vi "AR Drone - Gamepad NavData Video.vi"() -> (2 "Hover?":bool, 3 "Video Stream":picture)   [LabVIEW 2015]
doc: "Example demonstrating how to control the AR Drone with a joystick or gamepad and simultaneously receive navigation and video data."
uses:
  <vilib>/LVH/AR Drone Toolkit/Decode NavData/Typedefs/NavData Demo.ctl
  <vilib>/LVH/AR Drone Toolkit/Type Defs/Flight Animations.ctl
  <vilib>/Utility/inputDevices.llb/closeJoystick.vi
  <vilib>/LVH/AR Drone Toolkit/AR Drone.lvlib
panel:
  out "Pitching speed":dbl
  out "Yawing speed":sgl
  out "Vertical speed":sgl
  in  "Autopilot":bool
  in  "Stop FSM":bool
  in  "Reset":bool
  in  "Start":bool
  in  "Desired yaw":i16
  in  "Restart":bool
  in  "State":i8=1 min=1 max=33 step=1
  out "Downward loop":i8
  out "Snake loop":i8
  out "Upward loop":i8
  out "Current yaw":sgl
  out "Height":i16
  in  "Yaw speed":sgl(slide) min=-1 max=1 scale=-1.0..1.0
  in  "V speed":sgl(slide) min=-1 max=1 scale=-1.0..1.0
  in  "Pitch":sgl(slide) min=-1 max=1 scale=-1.0..1.0
  in  "Roll":sgl(slide) min=-1 max=1 scale=-1.0..1.0
  in  "display/gamepad":bool
  out "Gamepad Output":T1
  in  "Flight Animations":T2 items=["PHI_M30_DEG", "PHI_30_DEG", "THETA_M30_DEG", "THETA_30_DEG", "THETA_20DEG_YAW_200DEG", "THETA_20DEG_YAW_M2000DEG", "TURNAROUND", "TURNAROUND_GODOWN", "YAW_SHAKE", "YAW_DANCE", "PHI_DANCE", "THETA_DANCE", "VZ_DANCE", "WAVE", "PHI_THETA_MIXED", "DOUBLE_PHI_THETA_MIXED", "FLIP_AHEAD", "FLIP_BEHIND", "FLIP_LEFT", "FLIP_RIGHT", "NB_ANIM_MAYDAY"]
  out "NavData Out":T3
  out "Battery Remaining":dbl(slide) scale=0.0..100.0
  out "Axes Output":T4 {"Vertical Speed" scale=-1.0..1.0; "Yaw Speed" scale=-1.0..1.0; "Pitch" scale=-1.0..1.0; "Roll" scale=-1.0..1.0}
  in  "stop":bool
  # "Xbox Controller:\nLeft stick L/R - Roll\nLeft stick D/U - Pitch\nL/R Triggers - Vertical Speed\nRight stick L/R - Yaw Speed"
  # "Xbox Controller:\nA - take off\nB - emergency\nX - hover\nStart - Stop"
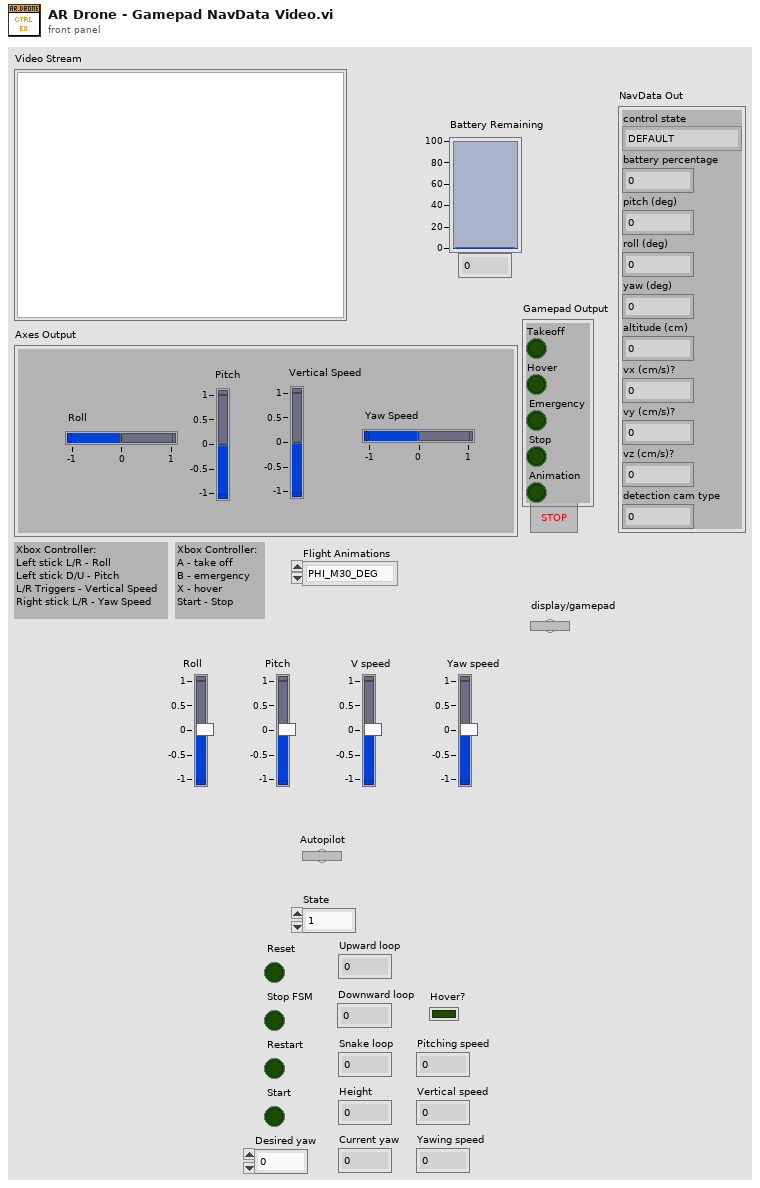
[diagram p1: front panel]
types:
  T1 = cluster{"Takeoff":bool, "Hover":bool, "Emergency":bool, "Stop":bool, "Animation":bool}
  T2 = typedef "AR Drone.lvlib/Flight Animations.ctl" = u16
  T3 = typedef "AR Drone.lvlib/NavData Demo.ctl" = cluster{"control state":enum32{"DEFAULT", "INIT", "LANDING", "FLYING", "HOVERING", "TEST", "TRANS_TAKEOFF", "TRANS_GOTOFIX", "TRANS_LANDING"}, "battery percentage":u32, "pitch (deg)":sgl, "roll (deg)":sgl, "yaw (deg)":sgl, "altitude (cm)":u32, "vx (cm/s)?":sgl, "vy (cm/s)?":sgl, "vz (cm/s)?":sgl, "detection cam type":u32}
  T4 = cluster{"Roll":dbl, "Pitch":dbl, "Vertical Speed":dbl, "Yaw Speed":dbl}
  T5 = typedef "AR Drone.lvlib/AR Drone Resource.ctl" = cluster{"UDP Control Connection":refnum<k16>, "UDP NavData Connection":refnum<k16>, "UDP Video Connection (Drone 1.0)":refnum<k16>, "TCP Video Connection (Drone 2.0)":refnum<k5>, "TCP Control Port Connection":refnum<k5>, "Drone IP address":string, "Drone Command Port":u16, "Drone NavData Port":u16, "Drone Vid Stream Port":u16, "Drone TCP Control Port":u16, "Home IP address":string, "Home Command Port":u16, "Home NavData Port":u16, "Home Vid Stream Port":u16, "Drone Version":i32}
  T6 = cluster{"Roll":sgl, "Pitch":sgl, "Vertical Speed":sgl, "Yaw Speed":sgl}
  T7 = cluster{"Roll":sgl, "Pitch":sgl, "V speed":sgl, "Yaw speed":sgl}
  T8 = cluster{"Yawing speed":sgl, "Pitching speed":dbl, "Vertical speed":sgl, "Yawing speed":sgl}
  T9 = cluster{"Roll":sgl, "Pitching speed":dbl, "V speed":sgl, "Yaw speed":sgl}
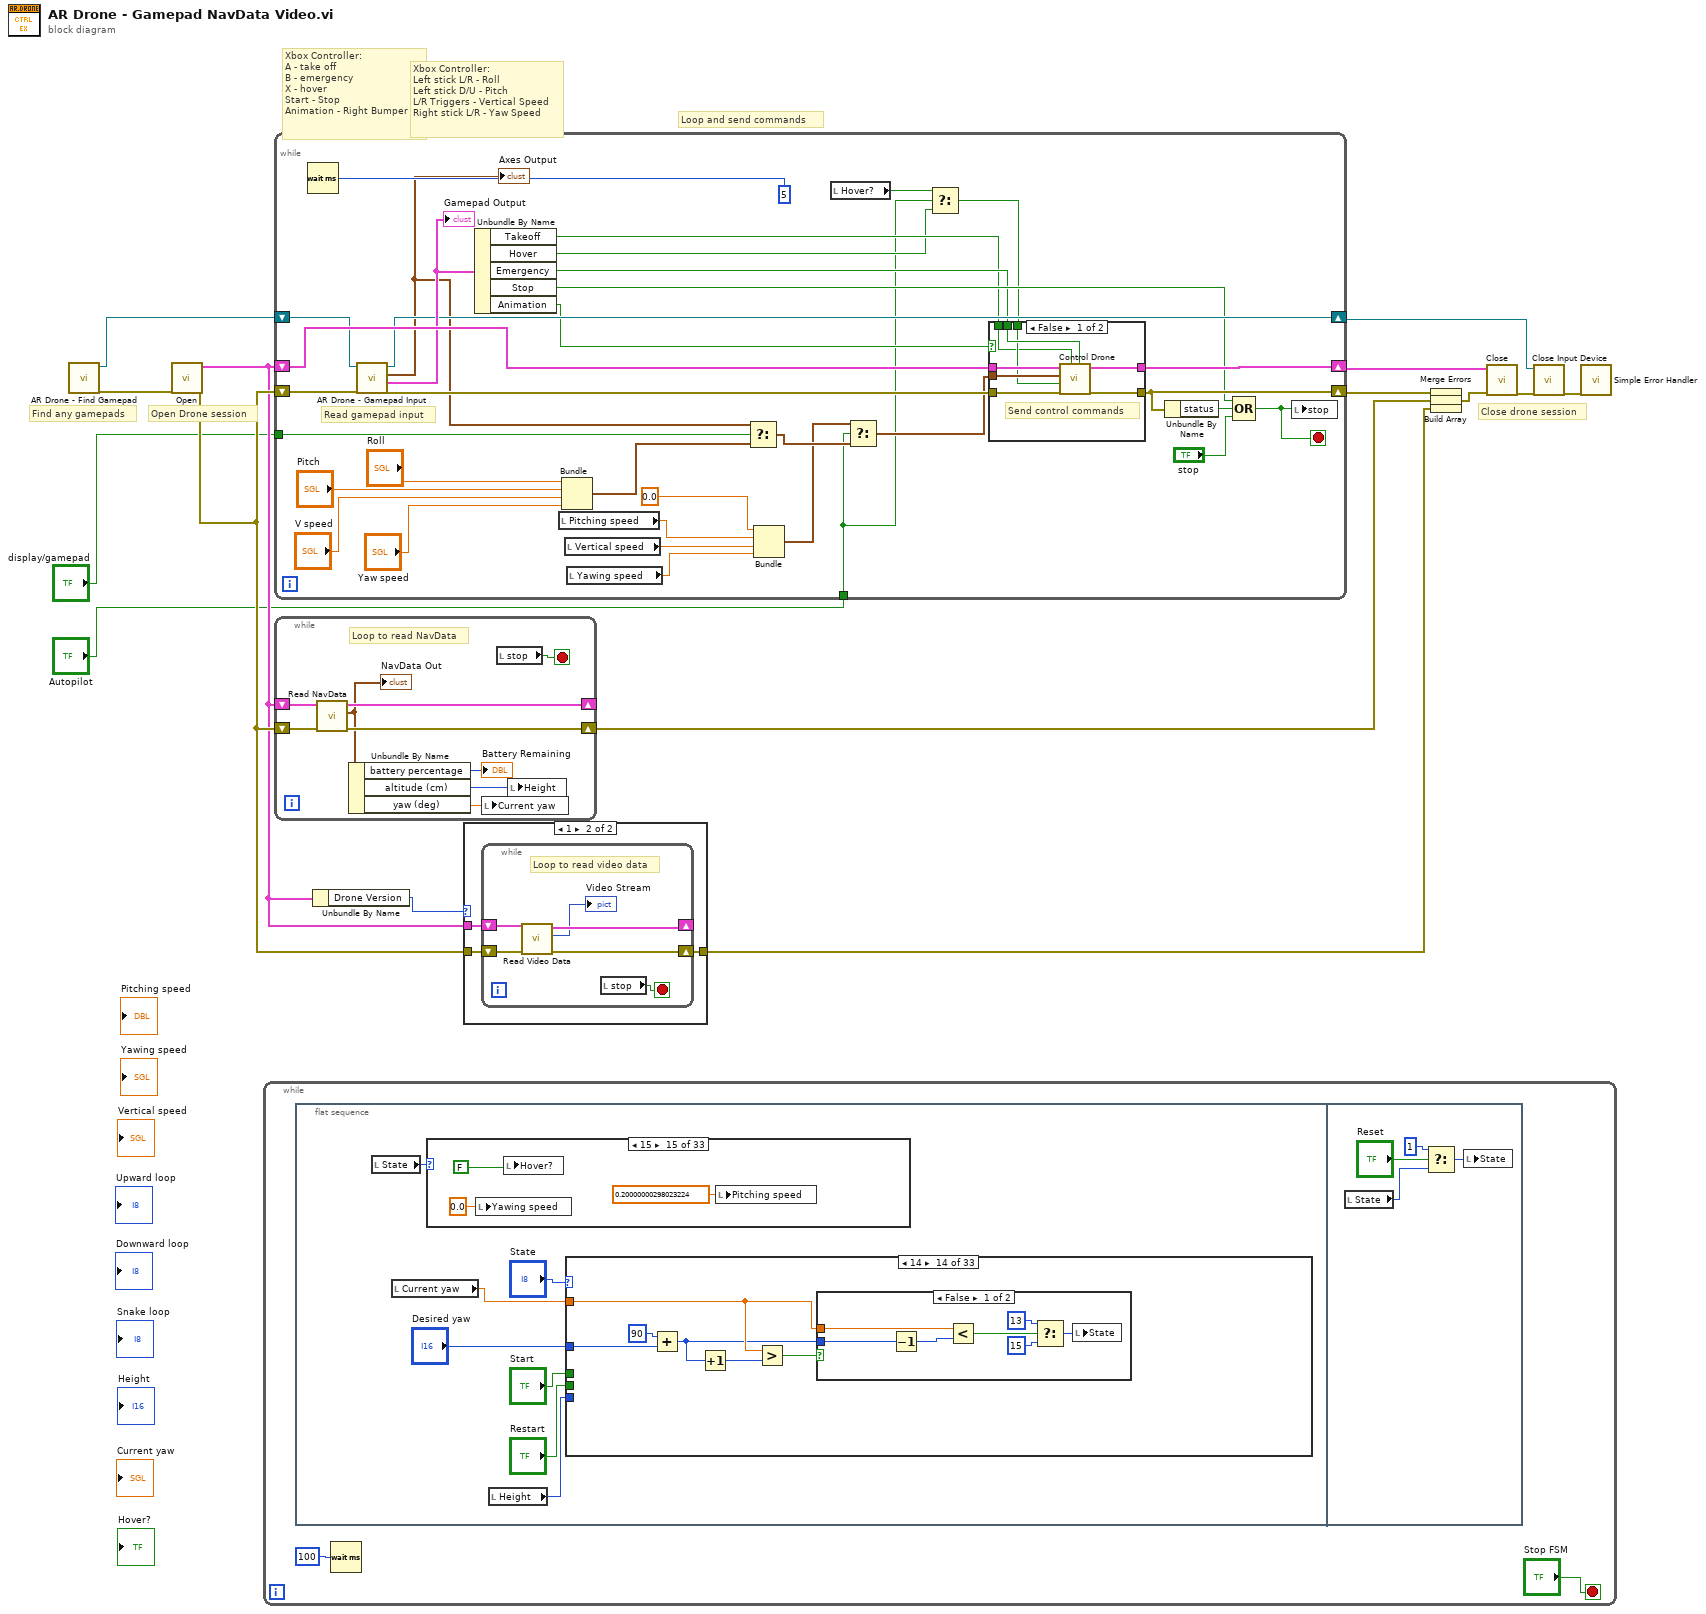
[diagram p0: block diagram]
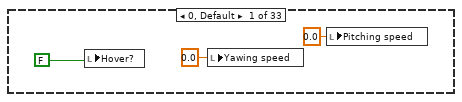
[diagram p2: hidden frame]
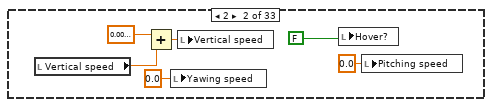
[diagram p3: hidden frame]
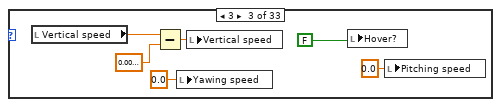
[diagram p4: hidden frame]
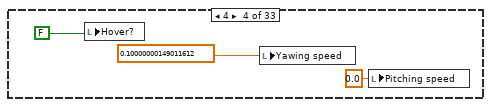
[diagram p5: hidden frame]
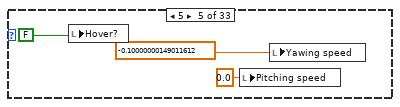
[diagram p6: hidden frame]
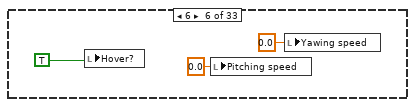
[diagram p7: hidden frame]
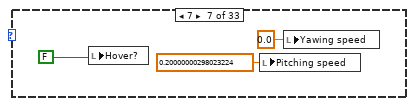
[diagram p8: hidden frame]
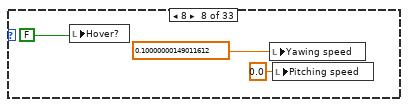
[diagram p9: hidden frame]
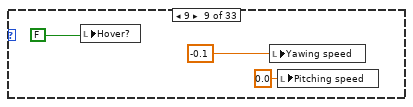
[diagram p10: hidden frame]
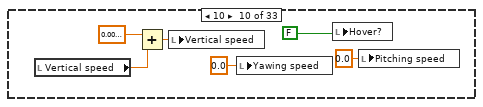
[diagram p11: hidden frame]
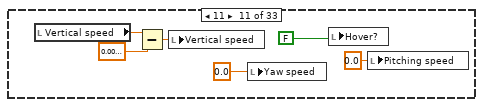
[diagram p12: hidden frame]
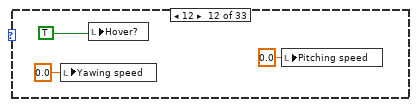
[diagram p13: hidden frame]
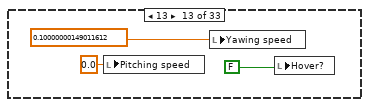
[diagram p14: hidden frame]
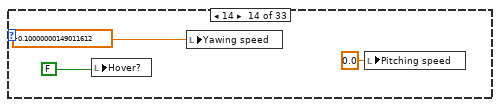
[diagram p15: hidden frame]
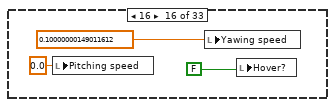
[diagram p16: hidden frame]
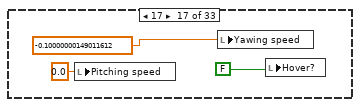
[diagram p17: hidden frame]
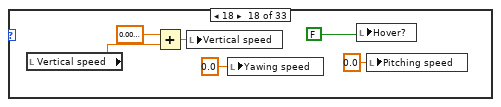
[diagram p18: hidden frame]
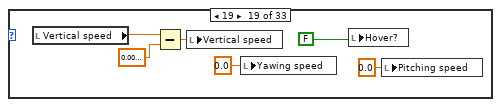
[diagram p19: hidden frame]
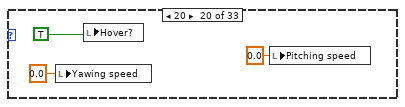
[diagram p20: hidden frame]
diagram:
  # "Loop and send commands"
  # "Close drone session"
  # "Open Drone session"
  # "Find any gamepads"
  # "Xbox Controller:\nLeft stick L/R - Roll\nLeft stick D/U - Pitch\nL/R Triggers - Vertical Speed\nRight stick L/R - Yaw Speed"
  # "Xbox Controller:\nA - take off\nB - emergency\nX - hover\nStart - Stop\nAnimation - Right Bumper"
  n1 = call "AR Drone - Find Gamepad.vi"() -> ("error out"=w11:errorcluster, "Refnum out"=w12:refnum<k1>)  [unwired: 10 in]
  n2 = call <vilib>:"Open.vi"("error in (no error)"=w11) -> ("error out"=w6:errorcluster, "AR Drone Resource"=w4:T5)  [unwired: 9 in]
  n3 = while {
    stop <- "Stop FSM" stop-if-true
    n4 = flat-sequence {
      frame #0 {
        n5 = local read "State"() -> (w20:i8)
        n6 = local read "Current yaw"() -> (w23:sgl)
        n7 = case shown="15" w20 {
          frame 0, Default {
            n8 = local write "Hover?"(FALSE) -> ()
            n9 = local write "Yawing speed"(sgl 0.0 ("Yawing speed")) -> ()
            n10 = local write "Pitching speed"(sgl 0.0 ("Yawing speed")) -> ()
          }
          frame 2 {
            n11 = local read "Vertical speed"() -> (w33:sgl)
            n12 = Add(x=sgl 0.01, y=w33) -> (x+y=w34:sgl)
            n13 = local write "Yawing speed"(sgl 0.0 ("Yawing speed")) -> ()
            n14 = local write "Vertical speed"(w34) -> ()
            n15 = local write "Hover?"(FALSE) -> ()
            n16 = local write "Pitching speed"(sgl 0.0 ("Yawing speed")) -> ()
          }
          frame 3 {
            n17 = local read "Vertical speed"() -> (w39:sgl)
            n18 = Subtract(x=w39, y=sgl 0.01 ("x")) -> (x-y=w40:sgl)
            n19 = local write "Yawing speed"(sgl 0.0 ("Yawing speed")) -> ()
            n20 = local write "Vertical speed"(w40) -> ()
            n21 = local write "Hover?"(FALSE) -> ()
            n22 = local write "Pitching speed"(sgl 0.0 ("Yawing speed")) -> ()
          }
          frame 4 {
            n23 = local write "Hover?"(FALSE) -> ()
            n24 = local write "Yawing speed"(sgl 0.1 ("Yawing speed")) -> ()
            n25 = local write "Pitching speed"(sgl 0.0 ("Yawing speed")) -> ()
          }
          frame 5 {
            n26 = local write "Hover?"(FALSE) -> ()
            n27 = local write "Pitching speed"(sgl 0.0 ("Yawing speed")) -> ()
            n28 = local write "Yawing speed"(sgl -0.1 ("Yawing speed")) -> ()
          }
          frame 6 {
            n29 = local write "Hover?"(TRUE) -> ()
            n30 = local write "Pitching speed"(sgl 0.0 ("Yawing speed")) -> ()
            n31 = local write "Yawing speed"(sgl 0.0 ("Yawing speed")) -> ()
          }
          frame 7 {
            n32 = local write "Hover?"(FALSE) -> ()
            n33 = local write "Pitching speed"(sgl 0.2 ("Yawing speed")) -> ()
            n34 = local write "Yawing speed"(sgl 0.0 ("Yawing speed")) -> ()
          }
          frame 8 {
            n35 = local write "Hover?"(FALSE) -> ()
            n36 = local write "Yawing speed"(sgl 0.1 ("Yawing speed")) -> ()
            n37 = local write "Pitching speed"(sgl 0.0 ("Yawing speed")) -> ()
          }
          frame 9 {
            n38 = local write "Hover?"(FALSE) -> ()
            n39 = local write "Yawing speed"(-0.1 ("Yawing speed")) -> ()
            n40 = local write "Pitching speed"(sgl 0.0 ("Yawing speed")) -> ()
          }
          frame 10 {
            n41 = local read "Vertical speed"() -> (w64:sgl)
            n42 = Add(x=sgl 0.01, y=w64) -> (x+y=w63:sgl)
            n43 = local write "Vertical speed"(w63) -> ()
            n44 = local write "Yawing speed"(sgl 0.0 ("Yawing speed")) -> ()
            n45 = local write "Hover?"(FALSE) -> ()
            n46 = local write "Pitching speed"(sgl 0.0 ("Yawing speed")) -> ()
          }
          frame 11 {
            n47 = local read "Vertical speed"() -> (w69:sgl)
            n48 = Subtract(x=w69, y=sgl 0.01) -> (x-y=w70:sgl)
            n49 = local write "Vertical speed"(w70) -> ()
            n50 = local write "Yaw speed"(sgl 0.0 ("Yawing speed")) -> ()
            n51 = local write "Hover?"(FALSE) -> ()
            n52 = local write "Pitching speed"(sgl 0.0 ("Yawing speed")) -> ()
          }
          frame 12 {
            n53 = local write "Yawing speed"(sgl 0.0 ("Yawing speed")) -> ()
            n54 = local write "Hover?"(TRUE) -> ()
            n55 = local write "Pitching speed"(sgl 0.0 ("Yawing speed")) -> ()
          }
          frame 13 {
            n56 = local write "Pitching speed"(sgl 0.0 ("Yawing speed")) -> ()
            n57 = local write "Yawing speed"(sgl 0.1 ("Yawing speed")) -> ()
            n58 = local write "Hover?"(FALSE) -> ()
          }
          frame 14 {
            n59 = local write "Hover?"(FALSE) -> ()
            n60 = local write "Yawing speed"(sgl -0.1 ("Yawing speed")) -> ()
            n61 = local write "Pitching speed"(sgl 0.0 ("Yawing speed")) -> ()
          }
          frame 15 {
            n62 = local write "Yawing speed"(sgl 0.0 ("Yawing speed")) -> ()
            n63 = local write "Hover?"(FALSE) -> ()
            n64 = local write "Pitching speed"(sgl 0.2 ("Yawing speed")) -> ()
          }
          frame 16 {
            n65 = local write "Pitching speed"(sgl 0.0 ("Yawing speed")) -> ()
            n66 = local write "Yawing speed"(sgl 0.1 ("Yawing speed")) -> ()
            n67 = local write "Hover?"(FALSE) -> ()
          }
          frame 17 {
            n68 = local write "Pitching speed"(sgl 0.0 ("Yawing speed")) -> ()
            n69 = local write "Yawing speed"(sgl -0.1 ("Yawing speed")) -> ()
            n70 = local write "Hover?"(FALSE) -> ()
          }
          frame 18 {
            n71 = local read "Vertical speed"() -> (w94:sgl)
            n72 = Add(x=sgl 0.01, y=w94) -> (x+y=w93:sgl)
            n73 = local write "Vertical speed"(w93) -> ()
            n74 = local write "Yawing speed"(sgl 0.0 ("Yawing speed")) -> ()
            n75 = local write "Hover?"(FALSE) -> ()
            n76 = local write "Pitching speed"(sgl 0.0 ("Yawing speed")) -> ()
          }
          frame 19 {
            n77 = local read "Vertical speed"() -> (w99:sgl)
            n78 = Subtract(x=w99, y=sgl 0.01) -> (x-y=w100:sgl)
            n79 = local write "Vertical speed"(w100) -> ()
            n80 = local write "Yawing speed"(sgl 0.0 ("Yawing speed")) -> ()
            n81 = local write "Hover?"(FALSE) -> ()
            n82 = local write "Pitching speed"(sgl 0.0 ("Yawing speed")) -> ()
          }
          frame 20 {
            n83 = local write "Yawing speed"(sgl 0.0 ("Yawing speed")) -> ()
            n84 = local write "Hover?"(TRUE) -> ()
            n85 = local write "Pitching speed"(sgl 0.0 ("Yawing speed")) -> ()
          }
          frame 21 {
            n86 = local write "Yawing speed"(sgl 0.0 ("Yawing speed")) -> ()
            n87 = local write "Hover?"(FALSE) -> ()
            n88 = local write "Pitching speed"(sgl 0.0 ("Yawing speed")) -> ()
          }
          frame 22 {
            n89 = local write "Pitching speed"(sgl 0.0 ("Yawing speed")) -> ()
            n90 = local write "Yawing speed"(sgl 0.1 ("Yawing speed")) -> ()
            n91 = local write "Hover?"(FALSE) -> ()
          }
          frame 23 {
            n92 = local write "Pitching speed"(sgl 0.0 ("Yawing speed")) -> ()
            n93 = local write "Yawing speed"(sgl -0.1 ("Yawing speed")) -> ()
            n94 = local write "Hover?"(FALSE) -> ()
          }
          frame 24 {
            n95 = local read "Vertical speed"() -> (w118:sgl)
            n96 = Add(x=sgl 0.01, y=w118) -> (x+y=w117:sgl)
            n97 = local write "Vertical speed"(w117) -> ()
            n98 = local write "Yawing speed"(sgl 0.0 ("Yawing speed")) -> ()
            n99 = local write "Hover?"(FALSE) -> ()
            n100 = local write "Pitching speed"(sgl 0.0 ("Yawing speed")) -> ()
          }
          frame 25 {
            n101 = local read "Vertical speed"() -> (w123:sgl)
            n102 = Subtract(x=w123, y=sgl 0.01) -> (x-y=w124:sgl)
            n103 = local write "Vertical speed"(w124) -> ()
            n104 = local write "Yawing speed"(sgl 0.0 ("Yawing speed")) -> ()
            n105 = local write "Hover?"(FALSE) -> ()
            n106 = local write "Pitching speed"(sgl 0.0 ("Yawing speed")) -> ()
          }
          frame 26 {
            n107 = local write "Yawing speed"(sgl 0.0 ("Yawing speed")) -> ()
            n108 = local write "Hover?"(TRUE) -> ()
            n109 = local write "Pitching speed"(sgl 0.0 ("Yawing speed")) -> ()
          }
          frame 27 {
            n110 = local write "Pitching speed"(sgl 0.0 ("Yawing speed")) -> ()
            n111 = local write "Yawing speed"(sgl 0.1 ("Yawing speed")) -> ()
            n112 = local write "Hover?"(FALSE) -> ()
          }
          frame 28 {
            n113 = local write "Pitching speed"(sgl 0.0 ("Yawing speed")) -> ()
            n114 = local write "Yawing speed"(sgl -0.1 ("Yawing speed")) -> ()
            n115 = local write "Hover?"(FALSE) -> ()
          }
          frame 29 {
            n116 = local write "Yawing speed"(sgl 0.0 ("Yawing speed")) -> ()
            n117 = local write "Hover?"(FALSE) -> ()
            n118 = local write "Pitching speed"(sgl 0.2 ("Yawing speed")) -> ()
          }
          frame 30 {
            n119 = local write "Pitching speed"(sgl 0.0 ("Yawing speed")) -> ()
            n120 = local write "Yawing speed"(sgl 0.1 ("Yawing speed")) -> ()
            n121 = local write "Hover?"(FALSE) -> ()
          }
          frame 31 {
            n122 = local write "Pitching speed"(sgl 0.0 ("Yawing speed")) -> ()
            n123 = local write "Yawing speed"(sgl -0.1 ("Yawing speed")) -> ()
            n124 = local write "Hover?"(FALSE) -> ()
          }
          frame 32 {
            n125 = local write "Yawing speed"(sgl 0.0 ("Yawing speed")) -> ()
            n126 = local write "Hover?"(TRUE) -> ()
            n127 = local write "Pitching speed"(sgl 0.0 ("Yawing speed")) -> ()
          }
          frame 33 {
            n128 = local write "Yawing speed"(sgl 0.0 ("Yawing speed")) -> ()
            n129 = local write "Hover?"(FALSE) -> ()
            n130 = local write "Pitching speed"(sgl 0.0 ("Yawing speed")) -> ()
          }
        }
        n131 = local read "Height"() -> (w24:i16)
        n132 = case shown="14" "State" {
          tunnel: "Start" -> [w152 _ _ _ _ _ _ _ _ _ _ _ _ _ _ _ _ _ _ _ _ _ _ _ _ _ _ _ _ _ _ _ _]
          tunnel: w24 -> [_ w156 w166 _ _ _ _ _ _ w226 w236 _ _ _ _ _ _ w309 w319 _ _ _ _ w359 w369 _ _ _ _ _ _ _ _]
          tunnel: w23 -> [_ _ _ w178 w189 _ _ w203 w215 _ _ _ w255 w269 _ w281 w295 _ _ _ _ w331 w345 _ _ _ w385 w399 _ w415 w429 _ _]
          tunnel: "Desired yaw" -> [_ _ _ w176 w188 _ _ w202 w214 _ _ _ w252 w268 _ w282 w296 _ _ _ _ w332 w346 _ _ _ w386 w400 _ w414 w428 _ _]
          tunnel: "Restart" -> [_ _ _ _ _ _ _ _ _ _ _ _ _ _ _ _ _ _ _ _ _ _ _ _ _ _ _ _ _ _ _ _ w453]
          frame Default {
            n133 = local write "Downward loop"(i8 5 ("pic loop 2")) -> ()
            n134 = Select(t=i8 2, s=w152, f=i8 1) -> (s? t:f=w155:i8)
            n135 = local write "Upward loop"(i8 5 ("pic loop")) -> ()
            n136 = local write "Snake loop"(i8 3 ("snake loop")) -> ()
            n137 = local write "State"(w155) -> ()
          }
          frame 2 {
            n138 = Greater?(x=w156, y=i16 152) -> (0:w157:bool)
            n139 = case shown="False" w157 {
              tunnel: w156 -> [w164 _]
              frame False {
                n140 = Less?(x=w164, y=i16 148) -> (x < y?=w162:bool)
                n141 = Select(t=i8 2, s=w162, f=i8 4) -> (s? t:f=w159:i8)
                n142 = local write "State"(w159) -> ()
              }
              frame True {
                n143 = local write "State"(i8 3 ("state")) -> ()
              }
            }
          }
          frame 3 {
            n144 = Greater?(x=w166, y=i16 152) -> (0:w168:bool)
            n145 = case shown="True" w168 {
              tunnel: w166 -> [w174 _]
              frame False {
                n146 = Less?(x=w174, y=i16 148) -> (x < y?=w172:bool)
                n147 = Select(t=i8 2, s=w172, f=i8 4) -> (s? t:f=w169:i8)
                n148 = local write "State"(w169) -> ()
              }
              frame True {
                n149 = local write "State"(i8 3 ("state")) -> ()
              }
            }
          }
          frame 4 {
            n150 = Increment(x=w176) -> (x+1=w177:i16)
            n151 = Greater?(x=w178, y=w177) -> (0:w179:bool)
            n152 = case shown="True" w179 {
              tunnel: w178 -> [w186 _]
              tunnel: w176 -> [w180 _]
              frame False {
                n153 = Decrement(x=w180) -> (x-1=w181:i16)
                n154 = Less?(x=w186, y=w181) -> (x < y?=w185:bool)
                n155 = Select(t=i8 4, s=w185, f=i8 6) -> (s? t:f=w182:i8)
                n156 = local write "State"(w182) -> ()
              }
              frame True {
                n157 = local write "State"(i8 5 ("state")) -> ()
              }
            }
          }
          frame 5 {
            n158 = Increment(x=w188) -> (x+1=w191:i16)
            n159 = Greater?(x=w189, y=w191) -> (0:w190:bool)
            n160 = case shown="False" w190 {
              tunnel: w189 -> [w198 _]
              tunnel: w188 -> [w192 _]
              frame False {
                n161 = Decrement(x=w192) -> (x-1=w193:i16)
                n162 = Less?(x=w198, y=w193) -> (x < y?=w197:bool)
                n163 = Select(t=i8 4, s=w197, f=i8 6) -> (s? t:f=w194:i8)
                n164 = local write "State"(w194) -> ()
              }
              frame True {
                n165 = local write "State"(i8 5 ("state")) -> ()
              }
            }
          }
          frame 6 {
            n166 = flat-sequence {
              frame #0 {
                n167 = call "Time Delay"() -> ()  [unwired: 11 in, 1 out]
              }
              frame #1 {
                n168 = local write "State"(i8 7 ("state")) -> ()
              }
            }
          }
          frame 7 {
            n169 = flat-sequence {
              frame #0 {
                n170 = call "Time Delay2"() -> ()  [unwired: 11 in, 1 out]
              }
              frame #1 {
                n171 = local write "State"(i8 8 ("state")) -> ()
              }
            }
          }
          frame 8 {
            n172 = Increment(x=w202) -> (x+1=w204:i16)
            n173 = Greater?(x=w203, y=w204) -> (0:w205:bool)
            n174 = case shown="False" w205 {
              tunnel: w203 -> [w212 _]
              tunnel: w202 -> [w206 _]
              frame False {
                n175 = Decrement(x=w206) -> (x-1=w207:i16)
                n176 = Less?(x=w212, y=w207) -> (x < y?=w211:bool)
                n177 = Select(t=i8 8, s=w211, f=i8 10) -> (s? t:f=w208:i8)
                n178 = local write "State"(w208) -> ()
              }
              frame True {
                n179 = local write "State"(i8 9 ("state")) -> ()
              }
            }
          }
          frame 9 {
            n180 = Increment(x=w214) -> (x+1=w217:i16)
            n181 = Greater?(x=w215, y=w217) -> (0:w216:bool)
            n182 = case shown="True" w216 {
              tunnel: w215 -> [w224 _]
              tunnel: w214 -> [w218 _]
              frame False {
                n183 = Decrement(x=w218) -> (x-1=w219:i16)
                n184 = Less?(x=w224, y=w219) -> (x < y?=w223:bool)
                n185 = Select(t=i8 8, s=w223, f=i8 10) -> (s? t:f=w220:i8)
                n186 = local write "State"(w220) -> ()
              }
              frame True {
                n187 = local write "State"(i8 9 ("state")) -> ()
              }
            }
          }
          frame 10 {
            n188 = Greater?(x=w226, y=i16 152) -> (0:w227:bool)
            n189 = case shown="False" w227 {
              tunnel: w226 -> [w234 _]
              frame False {
                n190 = Less?(x=w234, y=i16 148) -> (x < y?=w232:bool)
                n191 = Select(t=i8 10, s=w232, f=i8 12) -> (s? t:f=w229:i8)
                n192 = local write "State"(w229) -> ()
              }
              frame True {
                n193 = local write "State"(i8 11 ("state")) -> ()
              }
            }
          }
          frame 11 {
            n194 = Greater?(x=w236, y=i16 152) -> (0:w238:bool)
            n195 = case shown="False" w238 {
              tunnel: w236 -> [w244 _]
              frame False {
                n196 = Less?(x=w244, y=i16 148) -> (x < y?=w242:bool)
                n197 = Select(t=i8 10, s=w242, f=i8 12) -> (s? t:f=w239:i8)
                n198 = local write "State"(w239) -> ()
              }
              frame True {
                n199 = local write "State"(i8 11 ("state")) -> ()
              }
            }
          }
          frame 12 {
            n200 = flat-sequence {
              frame #0 {
                n201 = call "Time Delay3"() -> ()  [unwired: 11 in, 1 out]
              }
              frame #1 {
                n202 = local read "Upward loop"() -> (w250:i8)
                n203 = Decrement(x=w250) -> (x-1=w251:i8)
                n204 = local write "Upward loop"(w251) -> ()
                n205 = Equal To 0?(x=w251) -> (x = 0?=w246:bool)
                n206 = Select(t=i8 13, s=w246, f=i8 7) -> (s? t:f=w249:i8)
                n207 = local write "State"(w249) -> ()
              }
            }
          }
          frame 13 {
            n208 = Add(x=i16 90, y=w252) -> (x+y=w253:i16)
            n209 = Increment(x=w253) -> (x+1=w257:i16)
            n210 = Greater?(x=w255, y=w257) -> (0:w256:bool)
            n211 = case shown="True" w256 {
              tunnel: w255 -> [w264 _]
              tunnel: w253 -> [w258 _]
              frame False {
                n212 = Decrement(x=w258) -> (x-1=w259:i16)
                n213 = Less?(x=w264, y=w259) -> (x < y?=w263:bool)
                n214 = Select(t=i8 13, s=w263, f=i8 15) -> (s? t:f=w260:i8)
                n215 = local write "State"(w260) -> ()
              }
              frame True {
                n216 = local write "State"(i8 14 ("state")) -> ()
              }
            }
          }
          frame 14 {
            n217 = Add(x=i16 90, y=w268) -> (x+y=w267:i16)
            n218 = Increment(x=w267) -> (x+1=w270:i16)
            n219 = Greater?(x=w269, y=w270) -> (0:w271:bool)
            n220 = case shown="False" w271 {
              tunnel: w269 -> [w278 _]
              tunnel: w267 -> [w272 _]
              frame False {
                n221 = Decrement(x=w272) -> (x-1=w273:i16)
                n222 = Less?(x=w278, y=w273) -> (x < y?=w277:bool)
                n223 = Select(t=i8 13, s=w277, f=i8 15) -> (s? t:f=w274:i8)
                n224 = local write "State"(w274) -> ()
              }
              frame True {
                n225 = local write "State"(i8 14 ("state")) -> ()
              }
            }
          }
          frame 15 {
            n226 = flat-sequence {
              frame #0 {
                n227 = call "Time Delay4"() -> ()  [unwired: 11 in, 1 out]
              }
              frame #1 {
                n228 = local write "State"(i8 16 ("state")) -> ()
              }
            }
          }
          frame 16 {
            n229 = Add(x=i16 180, y=w282) -> (x+y=w286:i16)
            n230 = Increment(x=w286) -> (x+1=w283:i16)
            n231 = Greater?(x=w281, y=w283) -> (0:w284:bool)
            n232 = case shown="True" w284 {
              tunnel: w281 -> [w293 _]
              tunnel: w286 -> [w287 _]
              frame False {
                n233 = Decrement(x=w287) -> (x-1=w288:i16)
                n234 = Less?(x=w293, y=w288) -> (x < y?=w292:bool)
                n235 = Select(t=i8 16, s=w292, f=i8 18) -> (s? t:f=w289:i8)
                n236 = local write "State"(w289) -> ()
              }
              frame True {
                n237 = local write "State"(i8 17 ("state")) -> ()
              }
            }
          }
          frame 17 {
            n238 = Add(x=i16 180, y=w296) -> (x+y=w300:i16)
            n239 = Increment(x=w300) -> (x+1=w297:i16)
            n240 = Greater?(x=w295, y=w297) -> (0:w298:bool)
            n241 = case shown="True" w298 {
              tunnel: w295 -> [w307 _]
              tunnel: w300 -> [w301 _]
              frame False {
                n242 = Decrement(x=w301) -> (x-1=w302:i16)
                n243 = Less?(x=w307, y=w302) -> (x < y?=w306:bool)
                n244 = Select(t=i8 16, s=w306, f=i8 18) -> (s? t:f=w303:i8)
                n245 = local write "State"(w303) -> ()
              }
              frame True {
                n246 = local write "State"(i8 17 ("state")) -> ()
              }
            }
          }
          frame 18 {
            n247 = Greater?(x=w309, y=i16 152) -> (0:w311:bool)
            n248 = case shown="True" w311 {
              tunnel: w309 -> [w317 _]
              frame False {
                n249 = Less?(x=w317, y=i16 148) -> (x < y?=w315:bool)
                n250 = Select(t=i8 18, s=w315, f=i8 20) -> (s? t:f=w312:i8)
                n251 = local write "State"(w312) -> ()
              }
              frame True {
                n252 = local write "State"(i8 19 ("state")) -> ()
              }
            }
          }
          frame 19 {
            n253 = Greater?(x=w319, y=i16 152) -> (0:w321:bool)
            n254 = case shown="True" w321 {
              tunnel: w319 -> [w327 _]
              frame False {
                n255 = Less?(x=w327, y=i16 148) -> (x < y?=w325:bool)
                n256 = Select(t=i8 18, s=w325, f=i8 20) -> (s? t:f=w322:i8)
                n257 = local write "State"(w322) -> ()
              }
              frame True {
                n258 = local write "State"(i8 19 ("state")) -> ()
              }
            }
          }
          frame 20 {
            n259 = flat-sequence {
              frame #0 {
                n260 = call "Time Delay5"() -> ()  [unwired: 11 in, 1 out]
              }
              frame #1 {
                n261 = local write "State"(i8 21 ("state")) -> ()
              }
            }
          }
          frame 21 {
            n262 = flat-sequence {
              frame #0 {
                n263 = call "Time Delay6"() -> ()  [unwired: 11 in, 1 out]
              }
              frame #1 {
                n264 = local write "State"(i8 22 ("state")) -> ()
              }
            }
          }
          frame 22 {
            n265 = Add(x=i16 180, y=w332) -> (x+y=w333:i16)
            n266 = Increment(x=w333) -> (x+1=w336:i16)
            n267 = Greater?(x=w331, y=w336) -> (0:w335:bool)
            n268 = case shown="True" w335 {
              tunnel: w331 -> [w343 _]
              tunnel: w333 -> [w337 _]
              frame False {
                n269 = Decrement(x=w337) -> (x-1=w338:i16)
                n270 = Less?(x=w343, y=w338) -> (x < y?=w342:bool)
                n271 = Select(t=i8 22, s=w342, f=i8 24) -> (s? t:f=w339:i8)
                n272 = local write "State"(w339) -> ()
              }
              frame True {
                n273 = local write "State"(i8 23 ("state")) -> ()
              }
            }
          }
          frame 23 {
            n274 = Add(x=i16 180, y=w346) -> (x+y=w347:i16)
            n275 = Increment(x=w347) -> (x+1=w350:i16)
            n276 = Greater?(x=w345, y=w350) -> (0:w349:bool)
            n277 = case shown="True" w349 {
              tunnel: w345 -> [w357 _]
              tunnel: w347 -> [w351 _]
              frame False {
                n278 = Decrement(x=w351) -> (x-1=w352:i16)
                n279 = Less?(x=w357, y=w352) -> (x < y?=w356:bool)
                n280 = Select(t=i8 22, s=w356, f=i8 24) -> (s? t:f=w353:i8)
                n281 = local write "State"(w353) -> ()
              }
              frame True {
                n282 = local write "State"(i8 23 ("state")) -> ()
              }
            }
          }
          frame 24 {
            n283 = Greater?(x=w359, y=i16 152) -> (0:w360:bool)
            n284 = case shown="True" w360 {
              tunnel: w359 -> [w367 _]
              frame False {
                n285 = Less?(x=w367, y=i16 148) -> (x < y?=w365:bool)
                n286 = Select(t=i8 24, s=w365, f=i8 26) -> (s? t:f=w362:i8)
                n287 = local write "State"(w362) -> ()
              }
              frame True {
                n288 = local write "State"(i8 25 ("state")) -> ()
              }
            }
          }
          frame 25 {
            n289 = Greater?(x=w369, y=i16 152) -> (0:w370:bool)
            n290 = case shown="True" w370 {
              tunnel: w369 -> [w377 _]
              frame False {
                n291 = Less?(x=w377, y=i16 148) -> (x < y?=w375:bool)
                n292 = Select(t=i8 24, s=w375, f=i8 26) -> (s? t:f=w372:i8)
                n293 = local write "State"(w372) -> ()
              }
              frame True {
                n294 = local write "State"(i8 25 ("state")) -> ()
              }
            }
          }
          frame 26 {
            n295 = flat-sequence {
              frame #0 {
                n296 = call "Time Delay7"() -> ()  [unwired: 11 in, 1 out]
              }
              frame #1 {
                n297 = local read "Downward loop"() -> (w383:i8)
                n298 = Decrement(x=w383) -> (x-1=w384:i8)
                n299 = local write "Downward loop"(w384) -> ()
                n300 = Equal To 0?(x=w384) -> (x = 0?=w379:bool)
                n301 = Select(t=i8 27, s=w379, f=i8 21) -> (s? t:f=w382:i8)
                n302 = local write "State"(w382) -> ()
              }
            }
          }
          frame 27 {
            n303 = Add(x=i16 90, y=w386) -> (x+y=w390:i16)
            n304 = Increment(x=w390) -> (x+1=w387:i16)
            n305 = Greater?(x=w385, y=w387) -> (0:w388:bool)
            n306 = case shown="True" w388 {
              tunnel: w385 -> [w397 _]
              tunnel: w390 -> [w391 _]
              frame False {
                n307 = Decrement(x=w391) -> (x-1=w392:i16)
                n308 = Less?(x=w397, y=w392) -> (x < y?=w396:bool)
                n309 = Select(t=i8 27, s=w396, f=i8 29) -> (s? t:f=w393:i8)
                n310 = local write "State"(w393) -> ()
              }
              frame True {
                n311 = local write "State"(i8 28 ("state")) -> ()
              }
            }
          }
          frame 28 {
            n312 = Add(x=i16 90, y=w400) -> (x+y=w401:i16)
            n313 = Increment(x=w401) -> (x+1=w404:i16)
            n314 = Greater?(x=w399, y=w404) -> (0:w403:bool)
            n315 = case shown="False" w403 {
              tunnel: w399 -> [w411 _]
              tunnel: w401 -> [w405 _]
              frame False {
                n316 = Decrement(x=w405) -> (x-1=w406:i16)
                n317 = Less?(x=w411, y=w406) -> (x < y?=w410:bool)
                n318 = Select(t=i8 27, s=w410, f=i8 29) -> (s? t:f=w407:i8)
                n319 = local write "State"(w407) -> ()
              }
              frame True {
                n320 = local write "State"(i8 28 ("state")) -> ()
              }
            }
          }
          frame 29 {
            n321 = flat-sequence {
              frame #0 {
                n322 = call "Time Delay8"() -> ()  [unwired: 11 in, 1 out]
              }
              frame #1 {
                n323 = local write "State"(i8 30 ("state")) -> ()
              }
            }
          }
          frame 30 {
            n324 = Add(x=i16 180, y=w414) -> (x+y=w416:i16)
            n325 = Increment(x=w416) -> (x+1=w419:i16)
            n326 = Greater?(x=w415, y=w419) -> (0:w418:bool)
            n327 = case shown="True" w418 {
              tunnel: w415 -> [w426 _]
              tunnel: w416 -> [w420 _]
              frame False {
                n328 = Decrement(x=w420) -> (x-1=w421:i16)
                n329 = Less?(x=w426, y=w421) -> (x < y?=w425:bool)
                n330 = Select(t=i8 30, s=w425, f=i8 32) -> (s? t:f=w422:i8)
                n331 = local write "State"(w422) -> ()
              }
              frame True {
                n332 = local write "State"(i8 31 ("state")) -> ()
              }
            }
          }
          frame 31 {
            n333 = Add(x=i16 180, y=w428) -> (x+y=w430:i16)
            n334 = Increment(x=w430) -> (x+1=w433:i16)
            n335 = Greater?(x=w429, y=w433) -> (0:w432:bool)
            n336 = case shown="True" w432 {
              tunnel: w429 -> [w440 _]
              tunnel: w430 -> [w434 _]
              frame False {
                n337 = Decrement(x=w434) -> (x-1=w435:i16)
                n338 = Less?(x=w440, y=w435) -> (x < y?=w439:bool)
                n339 = Select(t=i8 30, s=w439, f=i8 32) -> (s? t:f=w436:i8)
                n340 = local write "State"(w436) -> ()
              }
              frame True {
                n341 = local write "State"(i8 31 ("state")) -> ()
              }
            }
          }
          frame 32 {
            n342 = flat-sequence {
              frame #0 {
                n343 = call "Time Delay9"() -> ()  [unwired: 11 in, 1 out]
              }
              frame #1 {
                n344 = local write "Downward loop"(i8 5 ("pic loop 2")) -> ()
                n345 = local write "Upward loop"(i8 5 ("pic loop 1")) -> ()
                n346 = local read "Snake loop"() -> (w446:i8)
                n347 = Decrement(x=w446) -> (x-1=w447:i8)
                n348 = Equal To 0?(x=w447) -> (x = 0?=w442:bool)
                n349 = local write "Snake loop"(w447) -> ()
                n350 = Select(t=i8 33, s=w442, f=i8 7) -> (s? t:f=w445:i8)
                n351 = local write "State"(w445) -> ()
              }
            }
          }
          frame 33 {
            n352 = Select(t=i8 1, s=w453, f=i8 33) -> (s? t:f=w452:i8)
            n353 = local write "State"(w452) -> ()
          }
        }
      }
      frame #1 {
        n354 = local read "State"() -> (w456:i8)
        n355 = Select(t=i8 1, s="Reset", f=w456) -> (s? t:f=w457:i8)
        n356 = local write "State"(w457) -> ()
      }
    }
    n357 = Wait (ms)(milliseconds to wait=u32 100) -> ()  [unwired: 1 out]
  }
  n358 = while {
    shift-right: [w490] -> w16
    shift-left: w4 -> [w491]
    shift-right: [w489] -> w9
    shift-left: w6 -> [w484]
    shift-right: [w481] -> w15
    shift-left: w12 -> [w485]
    tunnel: "display/gamepad" -> [w475]
    tunnel: "Autopilot" -> [w463]
    stop <- w477 stop-if-true
    # "Read gamepad input"
    n359 = Wait (ms)(milliseconds to wait=u32 5) -> ()  [unwired: 1 out]
    n360 = call "AR Drone - Gamepad Input.vi"("error in (no error)"=w484, "Refnum in"=w485) -> ("error out"=w483:errorcluster, "Gamepad Output"=w482:T1, "Control Cluster"=w474:T6, "Refnum out"=w481:refnum<k1>)  [unwired: 6 in]
    "Axes Output" <- w474
    "Gamepad Output" <- w482
    n361 = Unbundle By Name(w482) -> ("Takeoff"=w478:bool, "Hover"=w465:bool, "Emergency"=w479:bool, "Stop"=w480:bool, "Animation"=w476:bool)
    n362 = local read "Pitching speed"() -> (w462:dbl)
    n363 = Bundle("Roll"="Roll", "Pitch"="Pitch", "V speed"="V speed", "Yaw speed"="Yaw speed") -> (w470:T7)  [unwired: 1 in]
    n364 = local read "Vertical speed"() -> (w459:sgl)
    n365 = local read "Yawing speed"() -> (w460:sgl)
    n366 = Select(t=w474, s=w475, f=w470) -> (s? t:f=w468:T7)
    n367 = Bundle("Yawing speed"=sgl 0.0, "Pitching speed"=w462, "Vertical speed"=w459, "Yawing speed"=w460) -> (w458:T8)  [unwired: 1 in]
    n368 = local read "Hover?"() -> (w464:bool)
    n369 = Select(t=w458, s=w463, f=w468) -> (s? t:f=w467:T9)
    n370 = Select(t=w464, s=w463, f=w465) -> (s? t:f=w466:bool)
    n371 = case shown="False" w476 {
      tunnel: w491 -> [w499 w502]
      tunnel: [w498 w500] -> w490
      tunnel: [w497 w501] -> w489
      tunnel: w483 -> [w496 w503]
      tunnel: w467 -> [w495 _]
      tunnel: w479 -> [w494 _]
      tunnel: w466 -> [w493 _]
      tunnel: w478 -> [w492 _]
      frame False {
        # "Send control commands"
        n372 = call <vilib>:"Control Drone.vi"("Emergency Landing"=w494, "Takeoff/Land"=w492, "error in (no error)"=w496, "Hover"=w493, "Control Cluster"=w495, "AR Drone Resource"=w499) -> ("error out"=w497:errorcluster, "AR Drone Resource Out"=w498:T5)  [unwired: 4 in]
      }
      frame True {
        n373 = call <vilib>:"Execute Animation.vi"("error in (no error)"=w503, "Flight Animation"="Flight Animations", "AR Drone Resource"=w502) -> ("error out"=w501:errorcluster, "AR Drone Resource Out"=w500:T5)  [unwired: 7 in]
      }
    }
    n374 = Unbundle By Name(w489) -> ("status"=w487:bool)
    n375 = Compound Arithmetic op=OR(w480, w487, "stop") -> (w477:bool)
    n376 = local write "stop"(w477) -> ()
  }
  n377 = while {
    shift-right: [w512] -> _
    shift-left: w4 -> [w513]
    shift-right: [w510] -> w8
    shift-left: w6 -> [w511]
    stop <- w508 stop-if-true
    # "Loop to read NavData"
    n378 = call <vilib>:"Read NavData.vi"("error in (no error)"=w511, "AR Drone Resource"=w513) -> ("error out"=w510:errorcluster, "NavData Out"=w507:T3, "AR Drone Resource Out"=w512:T5)  [unwired: 7 in]
    "NavData Out" <- w507
    n379 = Unbundle By Name(w507) -> ("battery percentage"=→"Battery Remaining":u32, "altitude (cm)"=w506:u32, "yaw (deg)"=w505:sgl)
    n380 = local write "Current yaw"(w505) -> ()
    n381 = local read "stop"() -> (w508:bool)
    n382 = local write "Height"(w506) -> ()
  }
  n383 = Unbundle By Name(w4) -> ("Drone Version"=w3:i32)
  n384 = case shown="1" w3 {
    tunnel: w4 -> [_ w517]
    tunnel: [w514 w516] -> w7
    tunnel: w6 -> [w514 w515]
    frame 2, Default {
      # "If Drone 2.0, no streaming in line"
    }
    frame 1 {
      n385 = while {
        shift-right: [w521] -> _
        shift-left: w517 -> [w523]
        shift-right: [w520] -> w516
        shift-left: w515 -> [w522]
        stop <- w518 stop-if-true
        # "Loop to read video data"
        n386 = call <vilib>:"Read Video Data.vi"("error in (no error)"=w522, "AR Drone Resource"=w523) -> ("error out"=w520:errorcluster, "Video Stream"=→"Video Stream":picture, "AR Drone Resource Out"=w521:T5)  [unwired: 7 in]
        n387 = local read "stop"() -> (w518:bool)
      }
    }
  }
  n388 = Build Array(w9, w8, w7) -> (w5:errorcluster[])
  n389 = Merge Errors(w5) -> (w10:errorcluster)
  n390 = call <vilib>:"Close.vi"("error in (no error)"=w10, "AR Drone Resource"=w16) -> ("error out"=w14:errorcluster)  [unwired: 9 in]
  n391 = call-poly <vilib>:"Close Input Device.vi"("error in (no error)"=w14, "device ID"=w15) -> ("error out"=w13:errorcluster)  [unwired: 8 in]
  n392 = call <vilib>:"Simple Error Handler.vi"("error in (no error)"=w13) -> ()  [unwired: 4 in, 5 out]
